vi "inverse calibration function H2O.vi"(7 "x":dbl format="%#_13g") -> (8 "f_inv(x)":dbl)   [LabVIEW 2010, in "LicorLI7000.lvlib"]
uses:
  LicorLI7000.lvlib
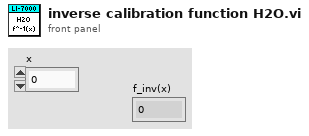
[diagram p1: front panel]
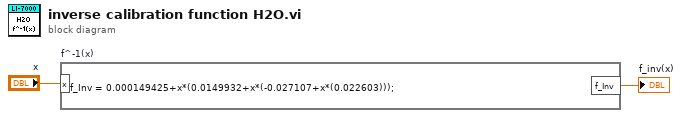
[diagram p0: block diagram]
diagram:
  n1 = formula code="f_Inv = 0.000149425+x*(0.0149932+x*(-0.027107+x*(0.022603)));" "f^-1(x)"("x"="x") -> ("f_Inv"=→"f_inv(x)":dbl)
